vi "Get Address.vi"() -> (3 "Enqueuer":refnum<class "Message Enqueuer.lvclass">)   [LabVIEW 2017, in "GlobalStopActor.lvclass"]
uses:
  GlobalStopActor.lvclass
  <vilib>/ActorFramework/Message Enqueuer/Message Enqueuer.lvclass
  C:/Program Files (x86)/National Instruments/LabVIEW 2017/vi.lib/ActorFramework/Actor/Actor.lvclass
  <vilib>/ActorFramework/Actor/Actor.lvclass
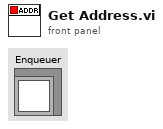
[diagram p1: front panel]
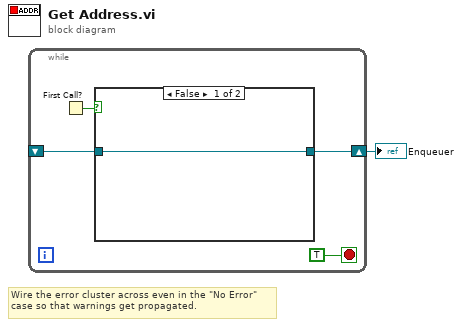
[diagram p0: block diagram]
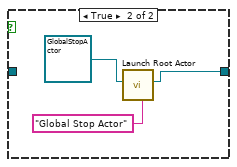
[diagram p2: hidden frame]
diagram:
  # "Wire the error cluster across even in the \"No Error\"\ncase so that warnings get propagated."
  n1 = while {
    shift-right: [w3] -> w1
    shift-left: _ -> [w2]
    stop <- TRUE stop-if-true
    n2 = First Call?() -> (First Call?: T/F=w5:bool)
    n3 = case shown="False" w5 {
      tunnel: [w6 w8] -> w3
      tunnel: w2 -> [w6 _]
      frame False {
      }
      frame True {
        n4 = call <vilib>:"Launch Root Actor.vi"("Debug Alias"="Global Stop Actor", "Actor"=refnum<class "GlobalStopActor.lvclass"> refnum ("GlobalStopActor.lvclass")) -> ("Actor's Enqueuer"=w8:refnum<class "Message Enqueuer.lvclass">)  [unwired: 8 in, 1 out]
      }
    }
  }
  "Enqueuer" <- w1
